vi "CanInit.vi"(9 "Baudrate":u16(ring)=1000 caption="K" items=["10"=10, "20"=20, "50"=50, "100"=100, "125"=125, "250"=250, "500"=500, "800"=800, "1000"=1000], 11 "CANPort":string(combo)="CAN1") -> (1 "GetStatus":T1={"baud"=1000, "acceptancemode"=1, "acceptancecode"=4294967295, "acceptancemask"=4294967294, "readtimeout"=3000, "writetimeout"=5000} {"acceptancecode" format="%x"; "acceptancemask" format="%x"})   [LabVIEW 2010]
panel:
  out "Error out":errorcluster {"code" format="%.0x"}
  in  "WriteTimeOut":u32=5000 caption="ms"
  in  "ReadTimeOut":u32=3000 caption="ms"
  in  "FilterMode":u32(ring)=1 items=["Dual ", "Single (default)"]
  in  "FilterMask":u32=4294967295 format="%x"
  in  "FilterCode":u32=4294967295 format="%x"
  # "输出："
  # "输入："
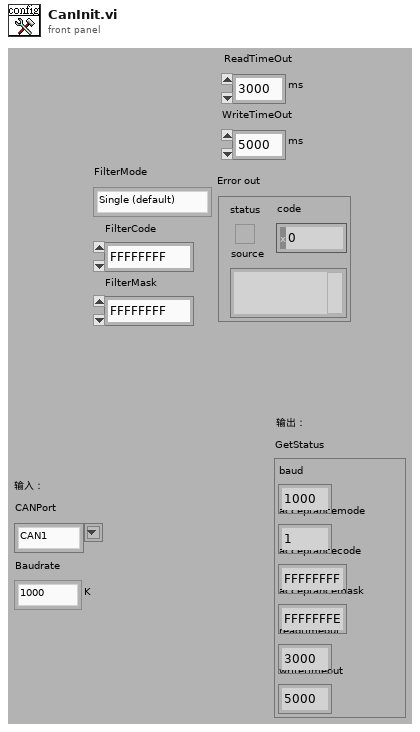
[diagram p1: front panel]
types:
  T1 = cluster{"baud":u32, "acceptancemode":u32, "acceptancecode":u32, "acceptancemask":u32, "readtimeout":u32, "writetimeout":u32}
  T2 = cluster{"baud":u32, "status":u32, "error_warning_limit":u32, "rx_errors":u32, "tx_errors":u32, "error_code":u32, "rx_buffer_size":u32, "rx_buffer_used":u32, "tx_buffer_size":u32, "tx_buffer_used":u32, "retval":u32, "type":u32, "acceptancecode":u32, "acceptancemask":u32, "acceptancemode":u32, "selfreception":u32, "readtimeout":u32, "writetimeout":u32}
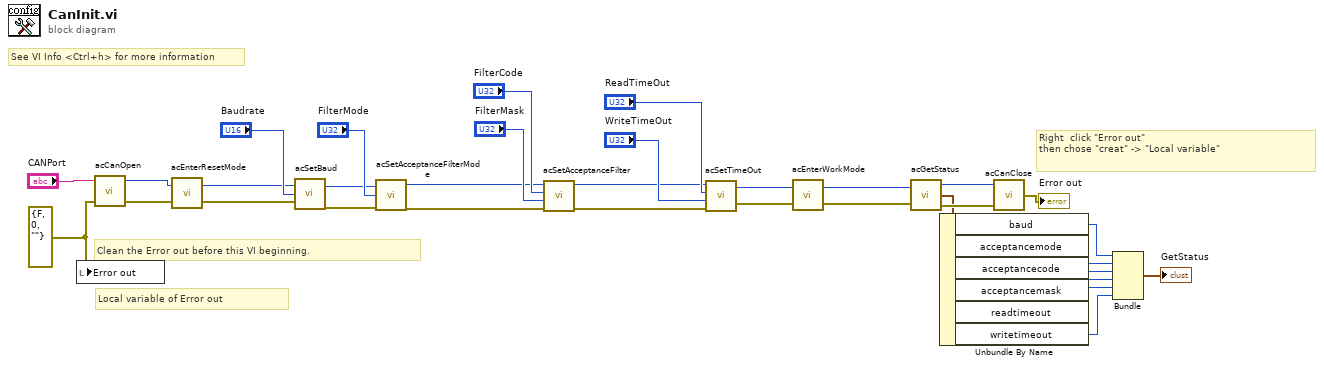
[diagram p0: block diagram]
diagram:
  w2 = errorcluster {"status"=FALSE, "code"=0, "source"=""} ("Error in")
  # "See VI Info <Ctrl+h> for more information"
  # "Right  click \"Error out\"\nthen chose \"creat\" -> \"Local variable\""
  # "Local variable of Error out"
  # "Clean the Error out before this VI beginning."
  n1 = local write "Error out"(w2) -> ()
  n2 = call "acCanOpen.vi"("Error in"=w2, "CANPort"="CANPort") -> ("Error out"=w4:errorcluster, "Handle"=w32:u32)  [unwired: 1 in, 1 out]
  n3 = call "acEnterResetMode.vi"("Error in"=w4, "Handle  in"=w32) -> ("Error out"=w1:errorcluster, "Handle out"=w5:u32)
  n4 = call "acSetBaud.vi"("Error in"=w1, "Baudrate"="Baudrate", "Handle  in"=w5) -> ("Error out"=w8:errorcluster, "Handle out"=w7:u32)
  n5 = call "acSetAcceptanceFilterMode.vi"("Error in"=w8, "FilterMode"="FilterMode", "Handle  in"=w7) -> ("Error out"=w26:errorcluster, "Handle out"=w25:u32)
  n6 = call "acSetAcceptanceFilter.vi"("Error in"=w26, "FilterMask"="FilterMask", "FilterCode"="FilterCode", "Handle  in"=w25) -> ("Error out"=w23:errorcluster, "Handle out"=w24:u32)
  n7 = call "acSetTimeOut.vi"("Error in"=w23, "WriteTimeOut"="WriteTimeOut", "Read TimeOut"="ReadTimeOut", "Handle  in"=w24) -> ("Error out"=w21:errorcluster, "Handle out"=w22:u32)
  n8 = call "acEnterWorkMode.vi"("Error in"=w21, "Handle  in"=w22) -> ("Error out"=w13:errorcluster, "Handle out"=w14:u32)
  n9 = call "acGetStatus.vi"("Handle  in"=w14, "Error in"=w13) -> ("Handle out"=w12:u32, "Status"=w10:T2, "Error out"=w11:errorcluster)
  n10 = Unbundle By Name "Unbundle By Name"(w10) -> ("baud"=w20:u32, "acceptancemode"=w19:u32, "acceptancecode"=w18:u32, "acceptancemask"=w17:u32, "readtimeout"=w16:u32, "writetimeout"=w15:u32)
  n11 = call "acCanClose.vi"("Error in"=w11, "Handle  in"=w12) -> ("Error out"=→"Error out":errorcluster)  [unwired: 1 in]
  n12 = Bundle "Bundle"("baud"=w20, "acceptancemode"=w19, "acceptancecode"=w18, "acceptancemask"=w17, "readtimeout"=w16, "writetimeout"=w15) -> (→"GetStatus":T1)  [unwired: 1 in]
